vi "WF3132 32Ch Multiplexer.vi"(2 "Packet (1)":u64, 4 "WF3132 I/O":T1={"FPGA I/O 1"="WF 3132/BankA", "FPGA I/O 2"="WF 3132/BankB", "FPGA I/O 3"="WF 3132/BankC", "FPGA I/O 4"="WF 3132/BankD"}) -> ()   [LabVIEW 2010]
doc: "This VI should be used together with the WF-3132 when creating a custom FPGA for VeriStand.\nIt uses one (1) packet."
uses:
  <vilib>/eio/EIONode/EIONode.xnode
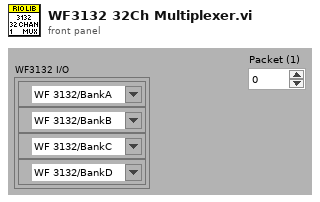
[diagram p1: front panel]
types:
  T1 = cluster{"FPGA I/O 1":refnum<k21>, "FPGA I/O 2":refnum<k21>, "FPGA I/O 3":refnum<k21>, "FPGA I/O 4":refnum<k21>}
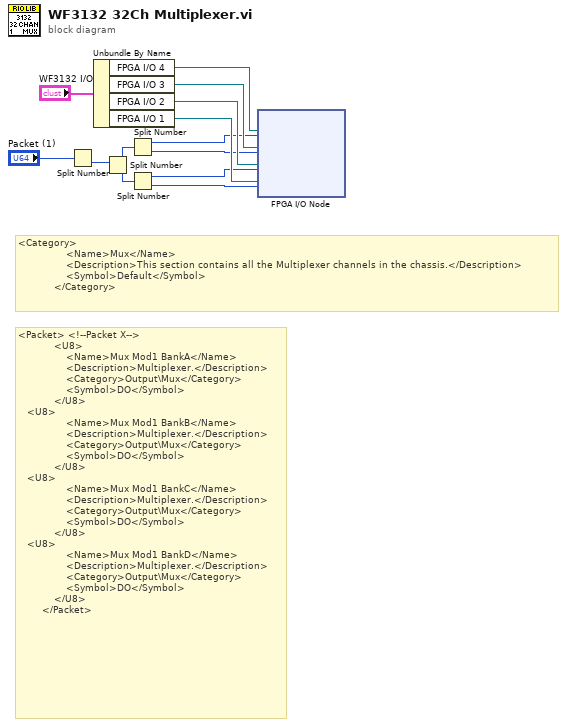
[diagram p0: block diagram]
diagram:
  # "<Category>\n                <Name>Mux</Name>\n                <Description>This section contains all the Multiplexer channels in the chassis.</Description>\n                <Symbol>Default</Symbol>\n            </Category>"
  # "<Packet>\t<!--Packet X-->\n            <U8>\n                <Name>Mux Mod1 BankA</Name>\n                <Description>Multiplexer.</Description>\n                <Category>Output\\Mux</Category>\n                <Symbol>DO</Symbol>\n            </U8>\n\t\t\t<U8>\n                <Name>Mux Mod1 BankB</Name>\n                <Description>Multiplexer.</Description>\n                <Category>Output\\Mux</Category>\n                <Symbol>DO</Symbol>\n            </U8>\n\t\t\t<U8>\n                <Name>Mux Mod1 BankC</Name>\n                <Description>Multiplexer.</Description>\n                <Category>Output\\Mux</Category>\n                <Symbol>DO</Symbol>\n            </U8>\n\t\t\t<U8>\n                <Name>Mux Mod1 BankD</Name>\n                <Description>Multiplexer.</Description>\n                <Category>Output\\Mux</Category>\n                <Symbol>DO</Symbol>\n            </U8>\n        </Packet>"
  n1 = Split Number(x="Packet (1)") -> (lo(x)=w6:u32)  [unwired: 1 out]
  n2 = Unbundle By Name("WF3132 I/O") -> ("FPGA I/O 4"=w12:refnum<k21>, "FPGA I/O 3"=w11:refnum<k21>, "FPGA I/O 2"=w10:refnum<k21>, "FPGA I/O 1"=w9:refnum<k21>)
  n3 = Split Number(x=w6) -> (hi(x)=w7:u16, lo(x)=w8:u16)
  n4 = Split Number(x=w7) -> (hi(x)=w4:u8, lo(x)=w3:u8)
  n5 = Split Number(x=w8) -> (hi(x)=w2:u8, lo(x)=w1:u8)
  n6 = xnode "FPGA I/O Node"("I/O Item"=w4, "FPGA I/O In"=w12, "I/O Item"=w3, "FPGA I/O In"=w11, "I/O Item"=w2, "FPGA I/O In"=w10, "I/O Item"=w1, "FPGA I/O In"=w9) -> ()  [unwired: 4 out]
